vi "Auto Functions.vi"(0 "VISA Resource Name":refnum<visa-resource-name>, 1 "Function (0: Auto Wide Reserve)":u16(ring) items=["Auto Wide Reserve ", "Auto Close Reserve", "Auto Sensitivity", "Auto Phase ", "Auto Null Offset"], 2 "Offset Quantity (0: CH1,X)":u16(ring) items=["CH1, X", "CH1, R [V]", "CH1, R [dBm]", "CH2, Y"], 5 "Error In (no error)":errorcluster) -> (14 "VISA Resource Name Out":refnum<visa-resource-name>, 19 "Error Out":errorcluster)   [LabVIEW 2010, in "Stanford Research 844.lvlib"]
doc: "This VI provides auto functions."
uses:
  <instrlib>/Stanford Research 844/Stanford Research 844.lvlib
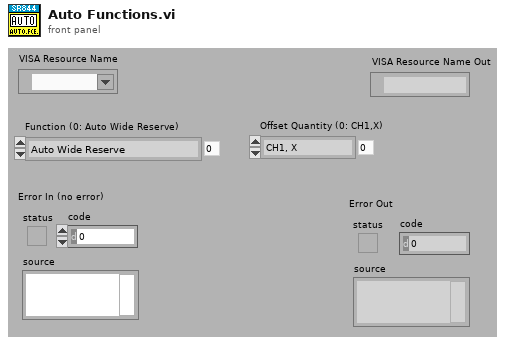
[diagram p1: front panel]
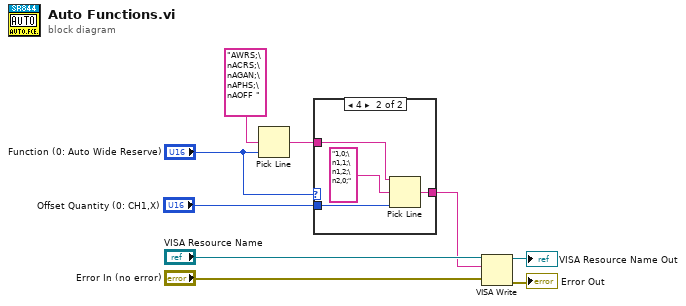
[diagram p0: block diagram]
diagram:
  n1 = Pick Line(multi-line string="AWRS;\nACRS;\nAGAN;\nAPHS;\nAOFF ", line index="Function (0: Auto Wide Reserve)") -> (output string=w2:string)  [unwired: 1 in]
  n2 = case shown="4" "Function (0: Auto Wide Reserve)" {
    tunnel: "Offset Quantity (0: CH1,X)" -> [_ w13]
    tunnel: w2 -> [w10 w12]
    tunnel: [w10 w11] -> w1
    frame 0, Default {
    }
    frame 4 {
      n3 = Pick Line(string ("")=w12, multi-line string="1,0;\n1,1;\n1,2;\n2,0;", line index=w13) -> (output string=w11:string)
    }
  }
  n4 = VISA Write(VISA resource name="VISA Resource Name", write buffer=w1, error in (no error)="Error In (no error)") -> (VISA resource name out=→"VISA Resource Name Out":refnum<visa-resource-name>, error out=→"Error Out":errorcluster)  [unwired: 1 out]
